vi "Unicode GB2312.vi"(2 "模式":enum16{"Unicode转GB2312", "GB2312转Unicode"}(ring), 7 "十六进制源码（不带0x标记）":string) -> (8 "转换后的编码":string)   [LabVIEW 2014]
panel:
  out "中文":string
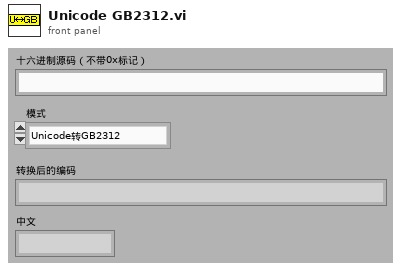
[diagram p1: front panel]
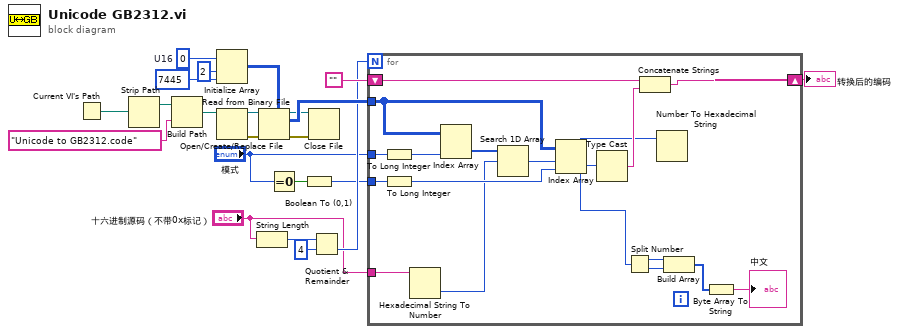
[diagram p0: block diagram]
diagram:
  w16 = u16 0  # U16
  n1 = Current VI's Path() -> (path=w22:path)
  n2 = Strip Path(path=w22) -> (stripped path=w21:path)  [unwired: 1 out]
  n3 = Build Path(base path=w21, name or relative path="Unicode to GB2312.code" ("名称或相对路径")) -> (appended path=w19:path)
  n4 = Initialize Array(w16, 2 ("维数大小"), 7445 ("维数大小")) -> (w13:u16[][])
  n5 = Open/Create/Replace File(file path (use dialog)=w19) -> (refnum out=w17:refnum<file>, error out=w18:errorcluster)  [unwired: 5 in, 1 out]
  n6 = String Length(string="十六进制源码（不带0x标记）") -> (length=w7:i32)
  n7 = Read from Binary File(5:w13, 8:w18, 11:w17) -> (0:w11:errorcluster, 2:w12:u16[][], 3:w10:refnum<file>)  [unwired: 3 in, 1 out]
  n8 = Equal To 0?(x="模式") -> (x = 0?=w2:bool)
  n9 = Boolean To (0,1)(Boolean=w2) -> (0, 1=w4:i16)
  n10 = Close File(refnum=w10, error in=w11) -> ()  [unwired: 2 out]
  n11 = Quotient & Remainder(x=w7, y=4) -> (floor(x/y)=w5:i32)  [unwired: 1 out]
  n12 = for {
    N: w5 -> [_]
    tunnel: w12 -> [w38]
    shift-right: [w35] -> w8
    shift-left: "" -> [w37]
    tunnel: w4 -> [w34]
    tunnel: "模式" -> [w33]
    tunnel: "十六进制源码（不带0x标记）" -> [w29]
    n13 = To Long Integer(number=w33) -> (32bit integer=w32:i32)
    n14 = To Long Integer(number=w34) -> (32bit integer=w31:i32)
    n15 = Hexadecimal String To Number(string=w29) -> (number=w28:u32)  [unwired: 2 in, 1 out]
    n16 = Index Array(array=w38, index (col)=w32) -> (element=w30:u16[])  [unwired: 1 in]
    n17 = Search 1D Array(1D array=w30, element=w28) -> (index of element=w39:i32)  [unwired: 1 in]
    n18 = Index Array(array=w38, index (row)=w39, index (col)=w31) -> (element=w25:u16)
    n19 = Type Cast(x=w25) -> (*(type *) &x=w36:string)  [unwired: 1 in]
    n20 = Split Number(x=w25) -> (hi(x)=w27:u8, lo(x)=w26:u8)
    n21 = Concatenate Strings(w37, w36) -> (w35:string)
    n22 = Number To Hexadecimal String(2:w25) -> ()  [unwired: 1 in, 1 out]
    n23 = Build Array(w27, w26) -> (w24:u8[])
    n24 = Byte Array To String(unsigned byte array=w24) -> (string=→"中文":string)
  }
  "转换后的编码" <- w8
